vi "Replace Class Constant.vi"(8 "error in (no error)":errorcluster, 10 "Constructor Method VI in":refnum<vi>, 11 "QControl Creation in":refnum<class "QControl Creation.lvclass">) -> (0 "error out":errorcluster, 2 "Constructor Method VI (dup)":refnum<vi>, 3 "QControl Creation (dup)":refnum<class "QControl Creation.lvclass">)   [LabVIEW 2015, in "QControl Creation.lvclass"]
doc: "<b> </b> <b> </b>\n©2016 Q Software Innovations, LLC (QSI)\nwritten by Quentin Alldredge\nproduced in LabVIEW 2015\n\nsupport@qsoftwareinnovations.com\nwww.qsoftwareinnovations.com\n\nAll rights reserved.\n\nRedistribution and use in source and binary forms, with or without modification, are permitted provided that the following conditions are met:\n\n * Redistributions of source code must retain the above copyright notice, this list of conditions and the following disclaimer.\n * Redistributions in binary form must reproduce the above copyright notice, this list of conditions and the following disclaimer in the documentation and/or other materials provided with the distribution.\n * Neither the name of Q Software Innovations, LLC. nor the names of its contributors may be used to endorse or promote products derived from this software without specific prior written permission.\n\nTHIS SOFTWARE IS PROVIDED BY THE COPYRIGHT HOLDERS AND CONTRIBUTORS \"AS IS\" AND ANY EXPRESS OR IMPLIED WARRANTIES, INCLUDING, BUT NOT LIMITED TO, THE IMPLIED WARRANTIES OF MERCHANTABILITY AND FITNESS FOR A PARTICULAR PURPOSE ARE DISCLAIMED. IN NO EVENT SHALL THE COPYRIGHT OWNER OR CONTRIBUTORS BE LIABLE FOR ANY DIRECT, INDIRECT, INCIDENTAL, SPECIAL, EXEMPLARY, OR CONSEQUENTIAL DAMAGES (INCLUDING, BUT NOT LIMITED TO, PROCUREMENT OF SUBSTITUTE GOODS OR SERVICES; LOSS OF USE, DATA, OR PROFITS; OR BUSINESS INTERRUPTION) HOWEVER CAUSED AND ON ANY THEORY OF LIABILITY, WHETHER IN CONTRACT, STRICT LIABILITY, OR TORT (INCLUDING NEGLIGENCE OR OTHERWISE) ARISING IN ANY WAY OUT OF THE USE OF THIS SOFTWARE, EVEN IF ADVISED OF THE POSSIBILITY OF SUCH DAMAGE."
uses:
  QControl Creation.lvclass
  <vilib>/Utility/traverseref.llb/TRef TravTarget.ctl
  QControl Creation.lvclass/QControl Creation.ctl
  New QControl Info/New QControl Info.lvclass/New QControl Info.ctl
  New QControl Info/Read New Class Path.vi
  <vilib>/Utility/error.llb/Error Cluster From Error Code.vi
  <vilib>/ErrorRing/Error Ring.xnode
  <vilib>/Utility/traverseref.llb/VI Scripting - Traverse.lvlib
  New QControl Info/New QControl Info.lvclass
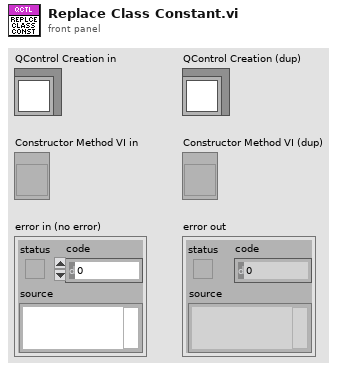
[diagram p1: front panel]
types:
  T1 = typedef "TRef TravTarget.ctl" = enum16{"FP", "BD", "Other"}
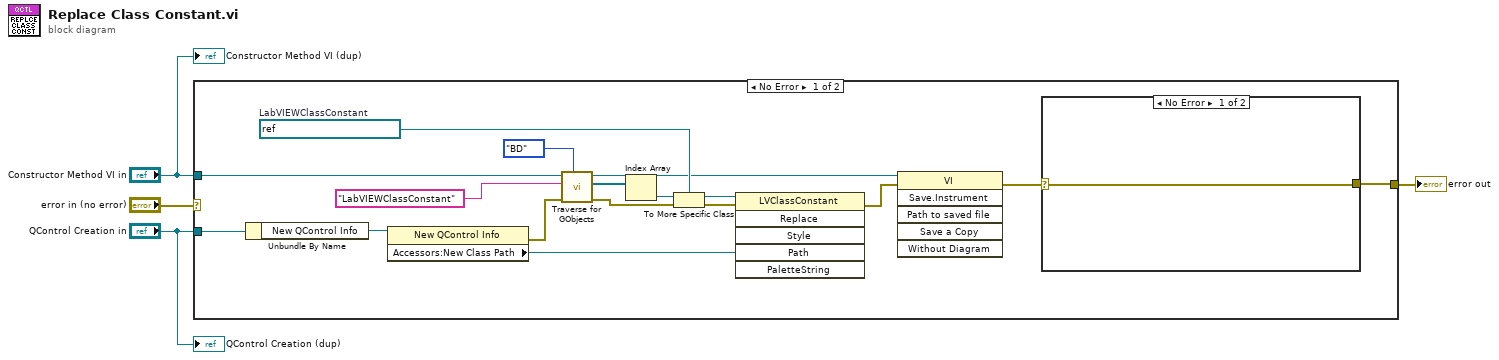
[diagram p0: block diagram]
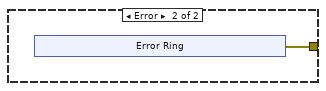
[diagram p2: hidden frame]
diagram:
  n1 = case shown="No Error" "error in (no error)" {
    selector: "error in (no error)" -> [_ w29]
    tunnel: [w7 w29] -> w3
    tunnel: "QControl Creation in" -> [w15 _]
    tunnel: "Constructor Method VI in" -> [w11 _]
    frame No Error {
      w17 = refnum<vi> refnum  # LabVIEWClassConstant
      n2 = Unbundle By Name(w15) -> ("New QControl Info"=w14:refnum<data-value>)
      n3 = property class="New QControl Info"(reference=w14) -> (error out=w5:errorcluster, "Accessors:New Class Path"=w6:path)  [unwired: 1 in, 1 out]
      n4 = call <vilib>:"Traverse for GObjects.vi"("Traverse Target"=TRef_TravTarget."BD", "error in (no error)"=w5, "Class Name"="LabVIEWClassConstant", "VI Refnum"=w11) -> ("error out"=w13:errorcluster, "References"=w19:refnum<vi>[], "dup VI Refnum"=w10:refnum<vi>)  [unwired: 4 in, 1 out]
      n5 = Index Array(array=w19) -> (element=w18:refnum<vi>)  [unwired: 1 in]
      n6 = To More Specific Class(target class=w17, reference=w18, error in=w13) -> (specific class reference=w16:refnum<vi>, error out=w12:errorcluster)
      n7 = invoke class="LVClassConstant" method="Replace"(reference=w16, error in=w12, "Path"=w6) -> (error out=w9:errorcluster)  [unwired: 3 in, 5 out]
      n8 = invoke class="VI" method="Save.Instrument"(reference=w10, error in=w9) -> (error out=w8:errorcluster)  [unwired: 4 in, 5 out]
      n9 = case shown="No Error" w8 {
        selector: w8 -> [w22 _]
        tunnel: [w22 w23] -> w7
        frame No Error {
        }
        frame Error {
          n10 = xnode "Error Ring"() -> ("error out"=w23:errorcluster)
        }
      }
    }
    frame Error {
    }
  }
  "error out" <- w3
  "QControl Creation (dup)" <- "QControl Creation in"
  "Constructor Method VI (dup)" <- "Constructor Method VI in"
